vi "CLK.vi"(2 "Reset":bool, 3 "Frequency [Hz]":dbl) -> (0 "Count":u32, 1 "Output":bool)   [LabVIEW 2022 SP3]
panel:
  out "Last":u32
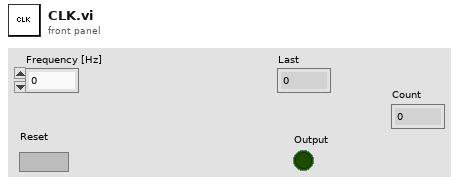
[diagram p1: front panel]
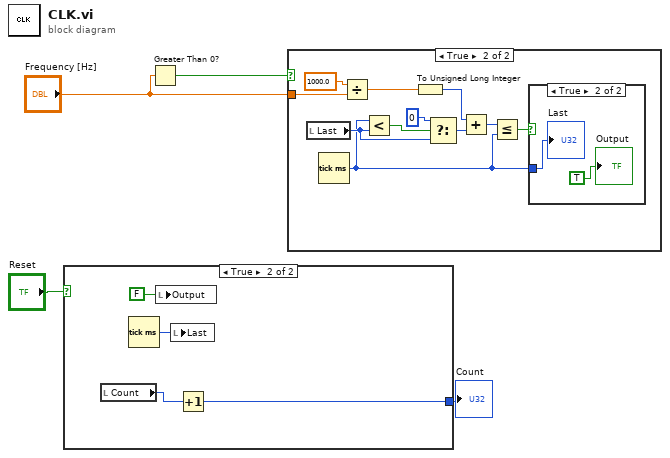
[diagram p0: block diagram]
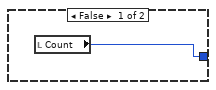
[diagram p2: hidden frame]
diagram:
  n1 = case shown="True" "Reset" {
    tunnel: [w5 w6] -> w1
    frame False {
      n2 = local read "Count"() -> (w5:u32)
    }
    frame True {
      n3 = local read "Count"() -> (w7:u32)
      n4 = Tick Count (ms)() -> (millisecond timer value=w8:u32)
      n5 = local write "Output"(FALSE ("Output")) -> ()
      n6 = local write "Last"(w8) -> ()
      n7 = Increment(x=w7) -> (x+1=w6:u32)
    }
  }
  "Count" <- w1
  n8 = Greater Than 0?(x="Frequency [Hz]") -> (x > 0?=w4:bool)
  n9 = case shown="True" w4 {
    tunnel: "Frequency [Hz]" -> [_ w19]
    frame False {
    }
    frame True {
      n10 = local read "Last"() -> (w16:u32)
      n11 = Tick Count (ms)() -> (millisecond timer value=w13:u32)
      n12 = Divide(x=1000.0, y=w19) -> (x/y=w12:dbl)
      n13 = Less?(x=w13, y=w16) -> (x < y?=w17:bool)
      n14 = To Unsigned Long Integer(number=w12) -> (unsigned 32bit integer=w11:u32)
      n15 = Select(t=u32 0, s=w17, f=w16) -> (s? t:f=w14:u32)
      n16 = Add(x=w11, y=w14) -> (x+y=w10:u32)
      n17 = Less Or Equal?(x=w10, y=w13) -> (x <= y?=w18:bool)
      n18 = case shown="True" w18 {
        tunnel: w13 -> [_ w21]
        frame False {
        }
        frame True {
          "Output" <- TRUE ("Output")
          "Last" <- w21
        }
      }
    }
  }
